vi "Fix Column Headings.vi"(1 "Column Headings":string[](array[string])=["Field", "Voltage1", "Voltage2", "Temperature", "Timestamp", "", "", "", "", "", "", "", "", "", "", "", "", "", ""], 2 "# Cols":i32=5) -> (0 "Column Headings":string[](array[string])=["Field", "Voltage1", "Voltage2", "Temperature", "Timestamp"])   [LabVIEW 2021]
doc: "This VI removes illegal characters from the column names and makes them valid variable names acceptable to most analysis software.\nScott Hannahs, NHMFL-FSU, February 1995"
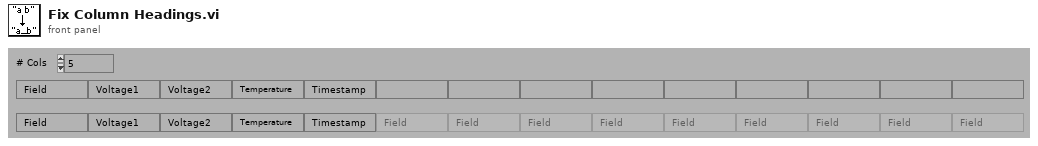
[diagram p1: front panel]
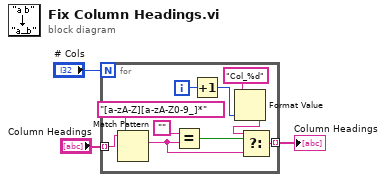
[diagram p0: block diagram]
diagram:
  n1 = for {
    N: "# Cols" -> [_]
    tunnel: "Column Headings" -> [w13] mode=indexing
    tunnel: [w11] -> w2 mode=indexing
    i -> [w6]
    n2 = Match Pattern(string=w13, regular expression="[a-zA-Z][a-zA-Z0-9_]*") -> (match substring=w10:string)  [unwired: 1 in, 3 out]
    n3 = Equal?(x="", y=w10) -> (x = y?=w8:bool)
    n4 = Increment(x=w6) -> (x+1=w4:i32)
    n5 = Format Value(format string="Col_%d", value (0)=w4) -> (output string=w7:string)  [unwired: 1 in]
    n6 = Select(t=w7, s=w8, f=w10) -> (s? t:f=w11:string)
  }
  "Column Headings" <- w2
